vi "Do Request.vi"(7 "Processing In":refnum<class "Processing.lvclass">, 11 "TestAuthController in":refnum<class "TestAuthController.lvclass">) -> (0 "error out":errorcluster, 5 "Processing":refnum<class "Processing.lvclass">)   [LabVIEW 2020, in "TestAuthController.lvclass"]
uses:
  TestAuthController.lvclass
  HTTP Server/Processing/Processing.lvclass
  HTTP Server/Processing/Processing.lvclass/Processing.ctl
  HTTP Server/Security/Security.lvclass
  TestUser/TestUser.lvclass
  4c2d0ac7-d900-4c3b-b536-e44d9f80a791.vi
  de48e8e9-b52e-4a0e-86b4-c4fb4766626b.vi
  3f6342d2-34d6-4d81-97dc-71330cffbf8f.vi
  9a42b769-e740-4a47-86af-88a39708e12e.vi
  4c2d0ac7-d900-4c3b-b536-e44d9f80a791.vi/9528e9df-aefc-4ce0-9221-106a337fd3b6.vi
  de48e8e9-b52e-4a0e-86b4-c4fb4766626b.vi/9528e9df-aefc-4ce0-9221-106a337fd3b6.vi
  3f6342d2-34d6-4d81-97dc-71330cffbf8f.vi/9528e9df-aefc-4ce0-9221-106a337fd3b6.vi
  9a42b769-e740-4a47-86af-88a39708e12e.vi/9528e9df-aefc-4ce0-9221-106a337fd3b6.vi
  <vilib>/IlluminatedG/IG HTTP Utils/HTTP Utils/Request/Get Target URI.vi
  <vilib>/IlluminatedG/lv-stream/URI/Get Path.vi
  HTTP Server/Values/Get Arg Map.vi
  <vilib>/Utility/error.llb/Error Cluster From Error Code.vi
  TestAuthController.lvclass/TestAuthController.ctl
  HTTP Server/HTTP Server.lvlib
  <vilib>/IlluminatedG/IG HTTP Utils/HTTP Utils/Response/Response.lvclass
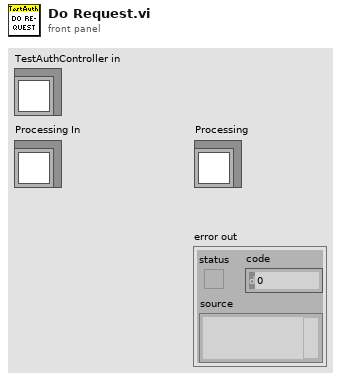
[diagram p1: front panel]
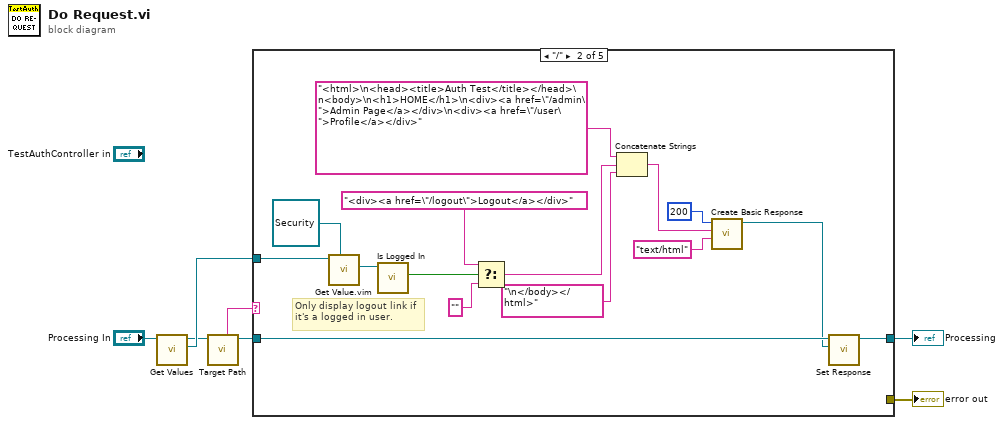
[diagram p0: block diagram]
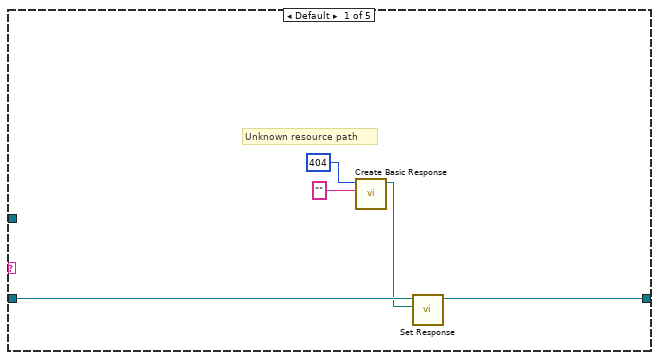
[diagram p2: hidden frame]
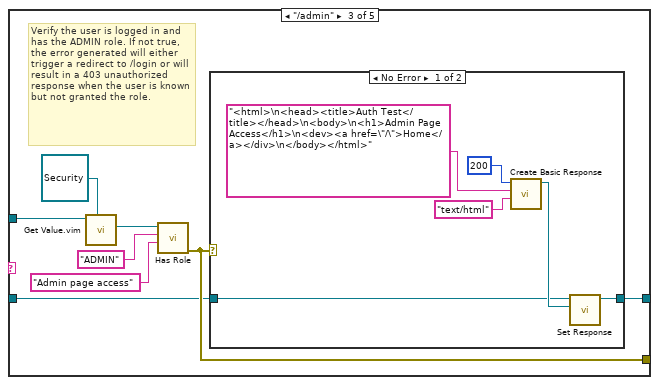
[diagram p3: hidden frame]
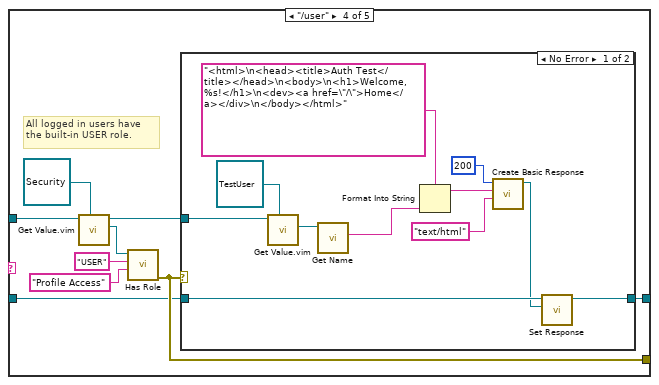
[diagram p5: hidden frame]
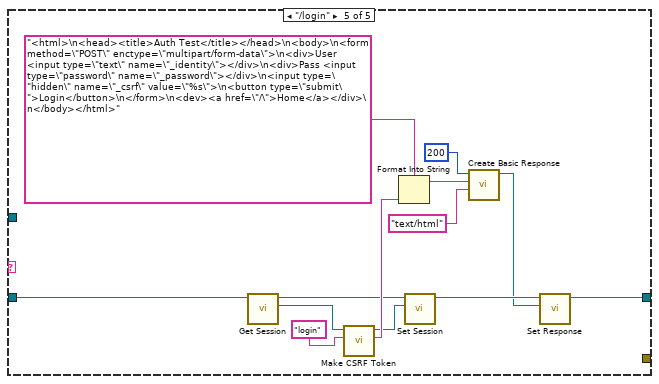
[diagram p7: hidden frame]
diagram:
  n1 = call "Get Values.vi"("Processing in"="Processing In") -> ("Values"=w5:refnum<class "Values.lvclass">, "Processing out"=w1:refnum<class "Processing.lvclass">)  [unwired: 9 in]
  n2 = call "Target Path.vi"("Processing in"=w1) -> ("Processing out"=w3:refnum<class "Processing.lvclass">, "Target Path"=w4:string)  [unwired: 9 in]
  n3 = case shown="\"/\"" w4 {
    tunnel: w5 -> [_ w25 w35 w51 _]
    tunnel: [_ _ w30 w45 _] -> w7
    tunnel: [w8 w15 w29 w43 w65] -> w2
    tunnel: w3 -> [w10 w14 w28 w44 w66]
    frame Default {
      # "Unknown resource path"
      n4 = call <vilib>:"Create Basic Response.vi"("Payload"="", "Status Code"=u16 404) -> ("Response out"=w9:refnum<class "Response.lvclass">)  [unwired: 8 in, 1 out]
      n5 = call "Set Response.vi"("Response"=w9, "Processing in"=w10) -> ("Processing out"=w8:refnum<class "Processing.lvclass">)  [unwired: 9 in]
    }
    frame "/" {
      # "Only display logout link if it's a logged in user."
      n6 = call "Get Value.vim"("Type / Server / Service (String)"=refnum<class "Security.lvclass"> refnum ("Security in"), "Arguments in"=w25) -> ("Value"=w17:refnum<class "Security.lvclass">)  [unwired: 7 in, 2 out]
      n7 = call "Is Logged In.vi"("Security in"=w17) -> ("Logged In"=w16:bool)  [unwired: 8 in, 2 out]
      n8 = Select(t="<div><a href=\"/logout\">Logout</a></div>", s=w16, f="") -> (s? t:f=w19:string)
      n9 = Concatenate Strings("<html>\n<head><title>Auth Test</title></head>\n<body>\n<h1>HOME</h1>\n<div><a href=\"/admin\">Admin Page</a></div>\n<div><a href=\"/user\">Profile</a></div>", w19, "\n</body></html>") -> (w22:string)
      n10 = call <vilib>:"Create Basic Response.vi"("Content-Type (text/plain)"="text/html", "Payload"=w22, "Status Code"=u16 200) -> ("Response out"=w13:refnum<class "Response.lvclass">)  [unwired: 7 in, 1 out]
      n11 = call "Set Response.vi"("Response"=w13, "Processing in"=w14) -> ("Processing out"=w15:refnum<class "Processing.lvclass">)  [unwired: 9 in]
    }
    frame "/admin" {
      # "Verify the user is logged in and has the ADMIN role. If not true, the error generated will either trigger a redirect to /login or will result in a 403 unauthorized response when the user is known but not granted the role."
      n12 = call "Get Value.vim"("Type / Server / Service (String)"=refnum<class "Security.lvclass"> refnum ("HTTP Server.lvlib:Security.lvclass"), "Arguments in"=w35) -> ("Value"=w33:refnum<class "Security.lvclass">)  [unwired: 7 in, 2 out]
      n13 = call "Has Role.vi"("Description (None)"="Admin page access", "Role"="ADMIN", "Security in"=w33) -> ("error out"=w30:errorcluster)  [unwired: 6 in, 2 out]
      n14 = case shown="No Error" w30 {
        tunnel: [w38 w42] -> w29
        tunnel: w28 -> [w36 w42]
        frame No Error {
          n15 = call <vilib>:"Create Basic Response.vi"("Content-Type (text/plain)"="text/html", "Payload"="<html>\n<head><title>Auth Test</title></head>\n<body>\n<h1>Admin Page Access</h1>\n<dev><a href=\"/\">Home</a></div>\n</body></html>", "Status Code"=u16 200) -> ("Response out"=w37:refnum<class "Response.lvclass">)  [unwired: 7 in, 1 out]
          n16 = call "Set Response.vi"("Response"=w37, "Processing in"=w36) -> ("Processing out"=w38:refnum<class "Processing.lvclass">)  [unwired: 9 in]
        }
        frame Error {
        }
      }
    }
    frame "/user" {
      # "All logged in users have the built-in USER role."
      n17 = call "Get Value.vim"("Type / Server / Service (String)"=refnum<class "Security.lvclass"> refnum ("HTTP Server.lvlib:Security.lvclass"), "Arguments in"=w51) -> ("Value"=w48:refnum<class "Security.lvclass">, "Arguments out"=w49:refnum<class "Values.lvclass">)  [unwired: 7 in, 1 out]
      n18 = call "Has Role.vi"("Description (None)"="Profile Access", "Role"="USER", "Security in"=w48) -> ("error out"=w45:errorcluster)  [unwired: 6 in, 2 out]
      n19 = case shown="No Error" w45 {
        tunnel: w49 -> [w56 _]
        tunnel: w44 -> [w54 w63]
        tunnel: [w52 w63] -> w43
        frame No Error {
          n20 = call "Get Value.vim"("Type / Server / Service (String)"=refnum<class "TestUser.lvclass"> refnum ("TestUser.lvclass"), "Arguments in"=w56) -> ("Value"=w55:refnum<class "TestUser.lvclass">)  [unwired: 7 in, 2 out]
          n21 = call "Get Name.vi"("TestUser in"=w55) -> ("Name"=w62:string)  [unwired: 8 in, 2 out]
          n22 = Format Into String(format string="<html>\n<head><title>Auth Test</title></head>\n<body>\n<h1>Welcome, %s!</h1>\n<dev><a href=\"/\">Home</a></div>\n</body></html>", w62) -> (resulting string=w61:string)  [unwired: 2 in, 1 out]
          n23 = call <vilib>:"Create Basic Response.vi"("Content-Type (text/plain)"="text/html", "Payload"=w61, "Status Code"=u16 200) -> ("Response out"=w53:refnum<class "Response.lvclass">)  [unwired: 7 in, 1 out]
          n24 = call "Set Response.vi"("Response"=w53, "Processing in"=w54) -> ("Processing out"=w52:refnum<class "Processing.lvclass">)  [unwired: 9 in]
        }
        frame Error {
        }
      }
    }
    frame "/login" {
      n25 = call "Get Session.vi"("Processing in"=w66) -> ("Session"=w70:refnum<class "Session.lvclass">, "Processing out"=w69:refnum<class "Processing.lvclass">)  [unwired: 9 in]
      n26 = call "Make CSRF Token.vi"("Token ID"="login", "Session In"=w70) -> ("Token"=w74:string, "Session"=w68:refnum<class "Session.lvclass">)  [unwired: 7 in, 1 out]
      n27 = Format Into String(format string="<html>\n<head><title>Auth Test</title></head>\n<body>\n<form method=\"POST\" enctype=\"multipart/form-data\">\n<div>User <input type=\"text\" name=\"_identity\"></div>\n<div>Pass <input type=\"password\" name=\"_password\"></div>\n<input type=\"hidden\" name=\"_csrf\" value=\"%s\">\n<button type=\"submit\">Login</button>\n</form>\n<dev><a href=\"/\">Home</a></div>\n</body></html>", w74) -> (resulting string=w73:string)  [unwired: 2 in, 1 out]
      n28 = call "Set Session.vi"("Session"=w68, "Processing in"=w69) -> ("Processing out"=w67:refnum<class "Processing.lvclass">)  [unwired: 9 in]
      n29 = call <vilib>:"Create Basic Response.vi"("Content-Type (text/plain)"="text/html", "Payload"=w73, "Status Code"=u16 200) -> ("Response out"=w64:refnum<class "Response.lvclass">)  [unwired: 7 in, 1 out]
      n30 = call "Set Response.vi"("Response"=w64, "Processing in"=w67) -> ("Processing out"=w65:refnum<class "Processing.lvclass">)  [unwired: 9 in]
    }
  }
  "error out" <- w7
  "Processing" <- w2
